vi "Set PID Values.vi"(8 "error in (no error)":errorcluster, 10 "PID":T1, 11 "Modbus Master in":refnum<class "Modbus Master.lvclass">) -> (0 "error out":errorcluster, 3 "Modbus Master out":refnum<class "Modbus Master.lvclass">)   [LabVIEW 2023, in "PIDModbus.lvlib"]
uses:
  PIDModbus.lvlib
  <vilib>/NI/Modbus Library/API/Master/Modbus Master.lvclass
  Controls/PID Cluster.ctl
  Controls/Register Enum.ctl
  <userlib>/_OpenG.lib/time/time.llb/openg_time.lvlib
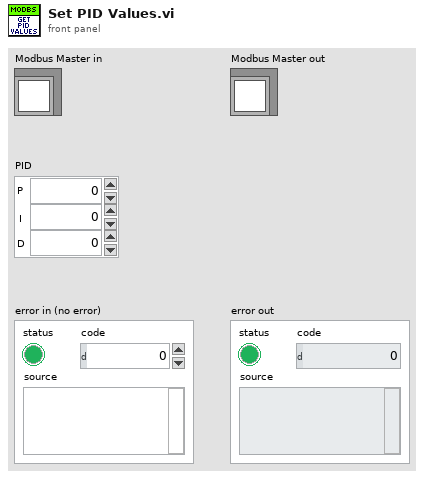
[diagram p1: front panel]
types:
  T1 = typedef "PIDModbus.lvlib/PID Cluster.ctl" = cluster{"P":u16, "I":u16, "D":u16}
  T2 = typedef "PIDModbus.lvlib/Register Enum.ctl" = u16
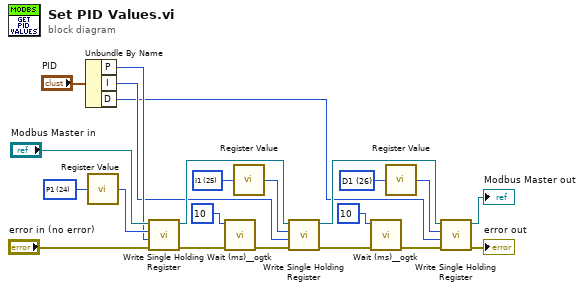
[diagram p0: block diagram]
diagram:
  w11 = T2 26 items=["PV"=0, "SV"=5, "P1"=24, "I1"=25, "D1"=26] ("Register")
  w16 = T2 25 items=["PV"=0, "SV"=5, "P1"=24, "I1"=25, "D1"=26] ("Register")
  w22 = T2 24 items=["PV"=0, "SV"=5, "P1"=24, "I1"=25, "D1"=26] ("Register")
  n1 = Unbundle By Name("PID") -> ("P"=w18:u16, "I"=w9:u16, "D"=w8:u16)
  n2 = call "Register Value.vi"("Register"=w22) -> ("RegAddr (Hex)"=w20:u16)
  n3 = call-dynamic "Write Single Holding Register.vi"("error in"="error in (no error)", "register to write"=w18, "address"=w20, "Modbus master in"="Modbus Master in") -> ("error out"=w17:errorcluster, "Modbus master out"=w14:refnum<class "Modbus Master.lvclass">)  [unwired: 6 in]
  n4 = call <userlib>:"Wait (ms)__ogtk.vi"("error in (no error)"=w17, "milliseconds to wait"=u32 10) -> ("error out"=w5:errorcluster)  [unwired: 8 in, 1 out]
  n5 = call "Register Value.vi"("Register"=w16) -> ("RegAddr (Hex)"=w15:u16)
  n6 = call-dynamic "Write Single Holding Register.vi"("error in"=w5, "register to write"=w9, "address"=w15, "Modbus master in"=w14) -> ("error out"=w2:errorcluster, "Modbus master out"=w13:refnum<class "Modbus Master.lvclass">)  [unwired: 6 in]
  n7 = call <userlib>:"Wait (ms)__ogtk.vi"("error in (no error)"=w2, "milliseconds to wait"=u32 10) -> ("error out"=w1:errorcluster)  [unwired: 8 in, 1 out]
  n8 = call "Register Value.vi"("Register"=w11) -> ("RegAddr (Hex)"=w10:u16)
  n9 = call-dynamic "Write Single Holding Register.vi"("error in"=w1, "register to write"=w8, "address"=w10, "Modbus master in"=w13) -> ("error out"=→"error out":errorcluster, "Modbus master out"=→"Modbus Master out":refnum<class "Modbus Master.lvclass">)  [unwired: 6 in]
